vi "Hold to Floor_Save Sweep Data to csv.vi"(0 "Test Information":T2={"Exp Name"="Cold Switching", "Lot"="0233A", "Wafer"="15", "Die Type"="L22", "Die X "="6", "Die Y"="8", "Exp"="1", "Die X_Y"="8"}, 1 "Filepath":path, 5 "Date Cluster":T3, 7 "Selected Exp Settings":T5={"Floor_Sweep_Stop_V"=36.0, "Resistance Threshold"=1.0, "Floor_Sweep_Start_V"=36.0, "Floor_Sweep_Step_V"=1.0, "Roof_Sweep_Stop_V"=36.0, "Roof_Sweep_Start_V"=36.0, "Roof_Sweep_Step_V"=1.0, "Experiment Name"="", "Meas_Type"=[0, 2, 4]}, 9 "ks5080A_Meaurements":T4, 11 "Cal Measurements":T7 {"Port 3 Capacitance" format="%#_6p"; "Port 2 Capacitance" format="%#_6p"; "Port 1 Capacitance" format="%#_6p"}, 12 "Additional Data":T8, 13 "Time":dbl[](array[numeric]), 14 "Meas Type":string="QuickView_") -> ()   [LabVIEW 2013]
uses:
  Controls/Date Control.ctl
  Controls/Test Information.ctl
  Controls/Additional Data.ctl
  Controls/ks5080A_Measurements.ctl
  Controls/Individual User Inputs_MultiTest.ctl
  Controls/Test Selection.ctl
  Controls/ENA_Marker Measurements.ctl
  <vilib>/Utility/file.llb/Write To Spreadsheet File (string).vi
panel:
  in  "Tab Control":T1(tab)
  # "Calculation Settings"
  # "Test Settings"
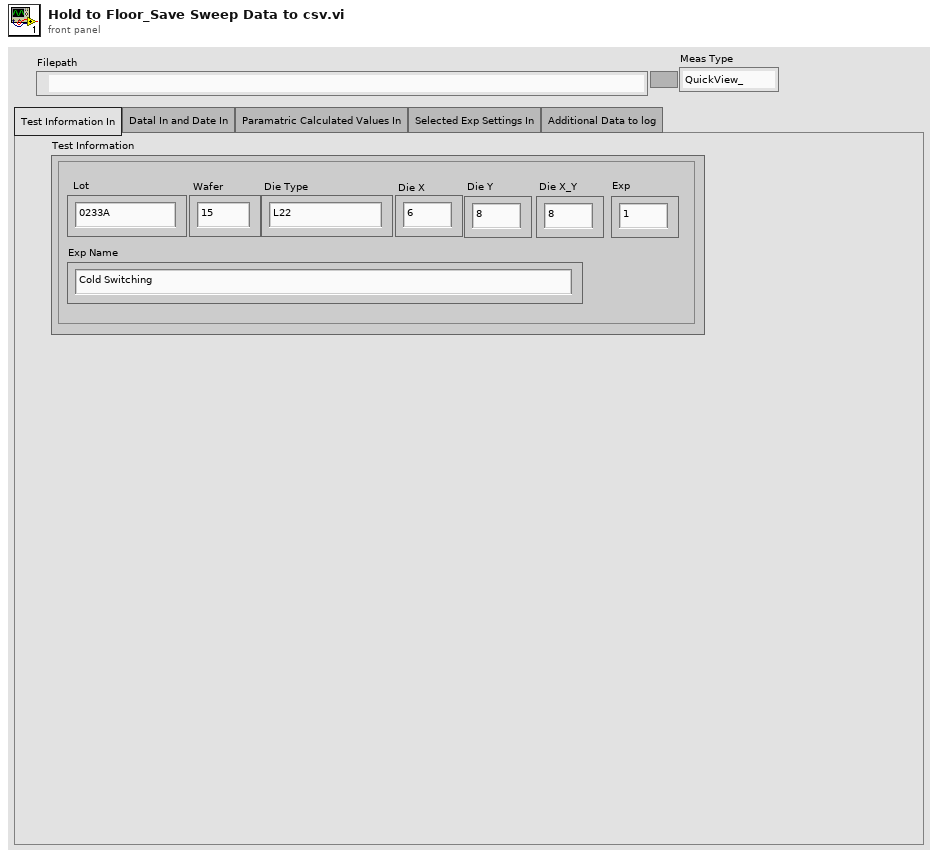
[diagram p1: front panel]
types:
  T1 = enum32{"Test Information In", "Datal In and Date In", "Paramatric Calculated Values In", "Selected Exp Settings In", "Additional Data to log"}
  T2 = typedef "Test Information.ctl" = cluster{"Exp Name":string, "Lot":string, "Wafer":string, "Die Type":string, "Die X ":string, "Die Y":string, "Exp":string, "Die X_Y":string}
  T3 = typedef "Date Control.ctl" = cluster{"Date":string, "Start Time":string, "Stop Time":string}
  T4 = typedef "ks5080A_Measurements.ctl" = cluster{"Bias_Sweep_Setting":dbl[], "Bias_voltage measurements":dbl[], "Bias_current measurements":dbl[], "P1_Capacitance":dbl[], "P2_Capacitance":dbl[], "DMM_Measurement_V":dbl[], "Contact_Source Current measurements":dbl[], "Contact_Sink Current measurements":dbl[], "Calculated_Resistance":dbl[], "P3_Capacitance":dbl[], "Port 1_S_parm":string[], "Port 2_S_parm":string[], "Port 3_S_parm":string[]}
  T5 = typedef "Individual User Inputs_MultiTest.ctl" = cluster{"Floor_Sweep_Stop_V":dbl, "Resistance Threshold":dbl, "Floor_Sweep_Start_V":dbl, "Floor_Sweep_Step_V":dbl, "Roof_Sweep_Stop_V":dbl, "Roof_Sweep_Start_V":dbl, "Roof_Sweep_Step_V":dbl, "Experiment Name":string, "Meas_Type":T6}
  T6 = typedef "Test Selection.ctl" = i32[]
  T7 = typedef "ENA_Marker Measurements.ctl" = cluster{"Port 1 Capacitance":dbl[], "Port 2 Capacitance":dbl[], "Port 3 Capacitance":dbl[], "Port 1_S_parm":string[], "Port 2_S_parm":string[], "Port 3_S_parm":string[]}
  T8 = typedef "Additional Data.ctl" = cluster{"P2_Capacitance_PostTest":dbl[], "P1_Capacitance _PostTest":dbl[], "P1_Capacitance_PreTest":dbl[], "P2_Capacitance_PreTest":dbl[]}
  T9 = enum16{"open", "replace", "create", "open or create", "replace or create", "replace or create with confirmation"}
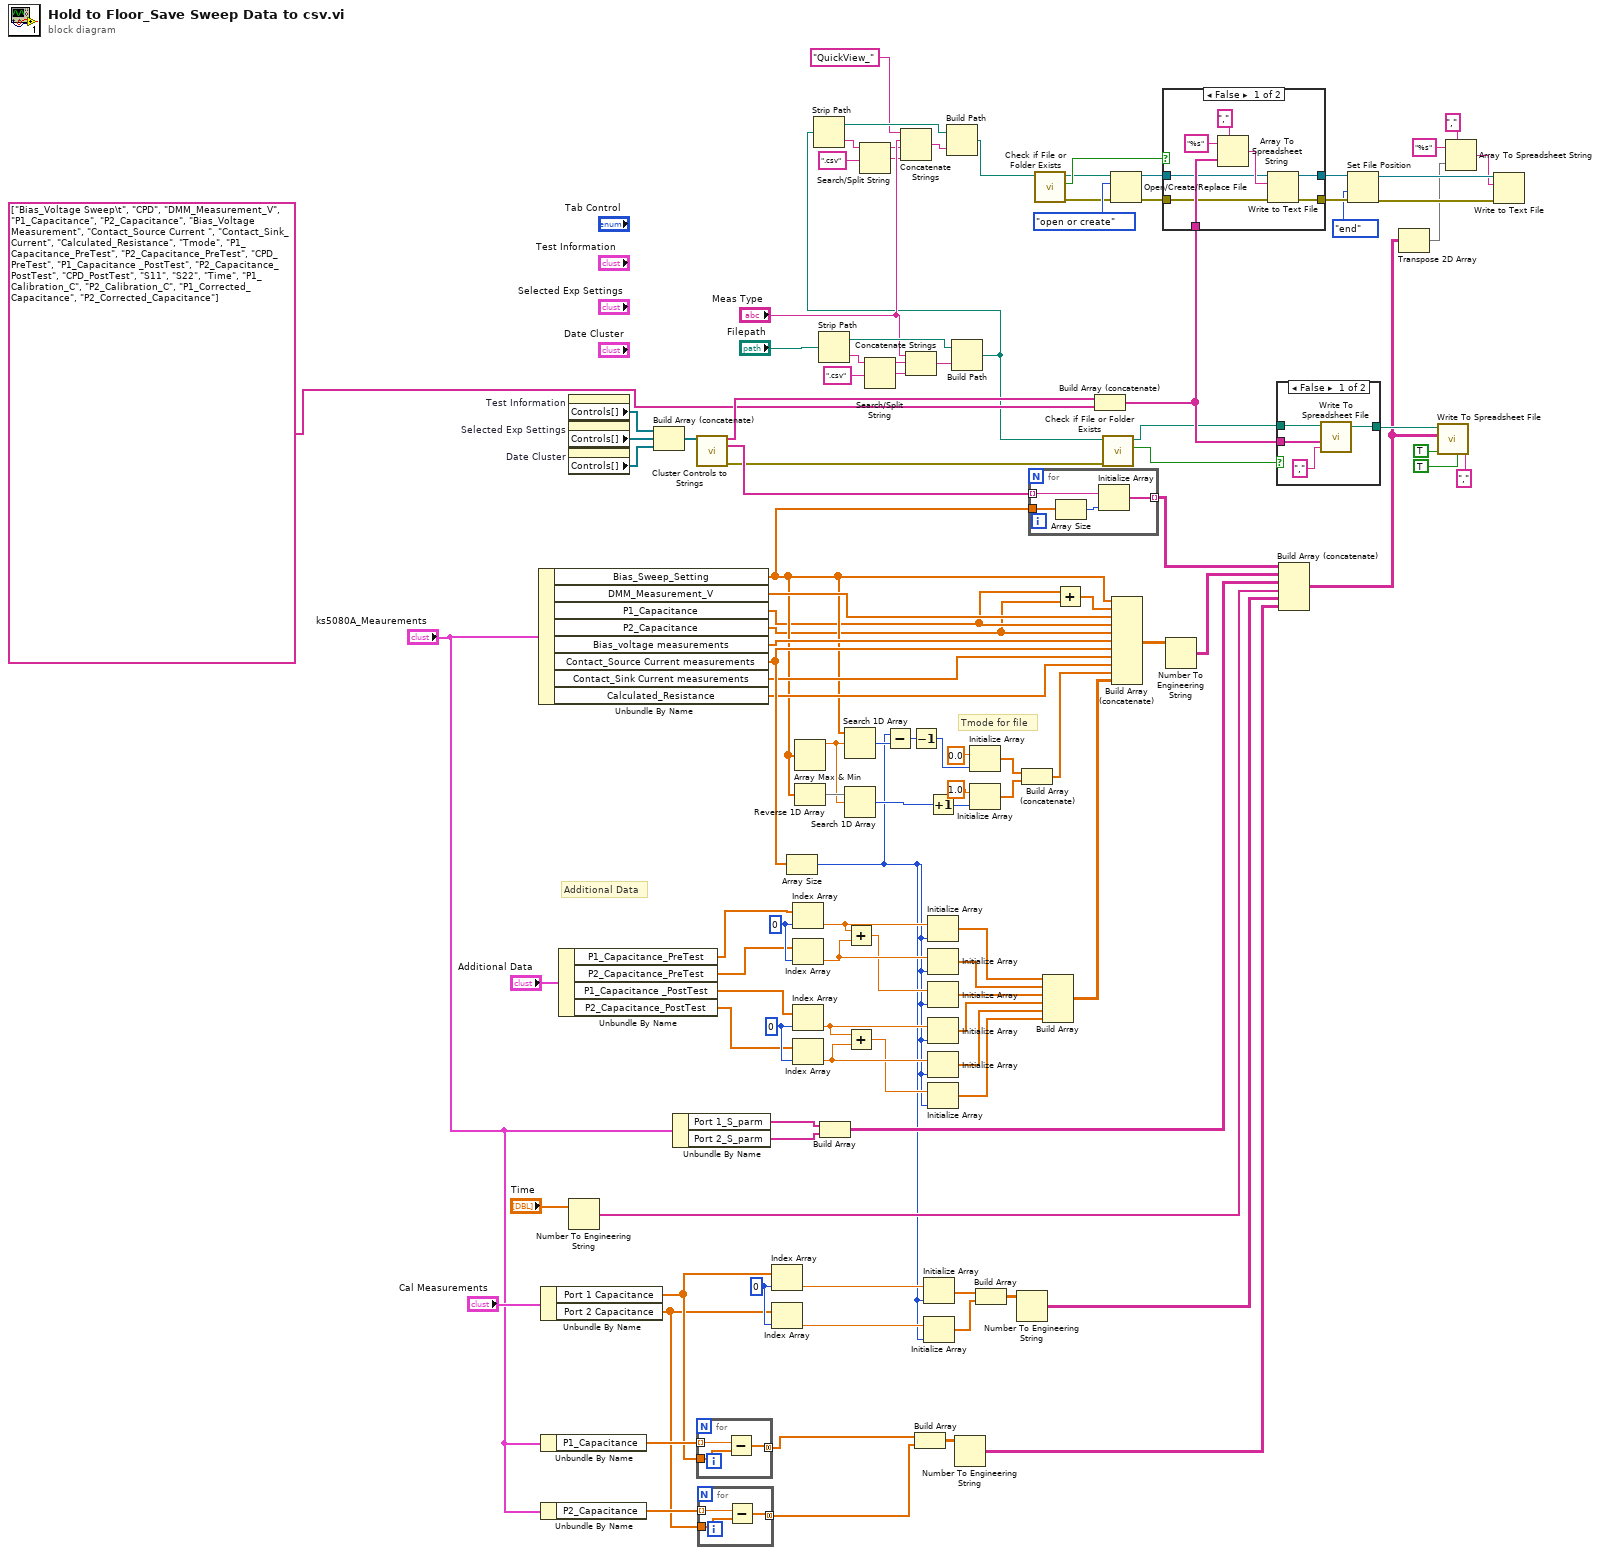
[diagram p0: block diagram]
diagram:
  w17 = 0 ("index")
  w98 = 0 ("index")
  w99 = 0 ("index")
  # "Tmode for file"
  # "Additional Data"
  n1 = Unbundle By Name("ks5080A_Meaurements") -> ("Bias_Sweep_Setting"=w23:dbl[], "DMM_Measurement_V"=w73:dbl[], "P1_Capacitance"=w21:dbl[], "P2_Capacitance"=w20:dbl[], "Bias_voltage measurements"=w72:dbl[], "Contact_Source Current measurements"=w71:dbl[], "Contact_Sink Current measurements"=w70:dbl[], "Calculated_Resistance"=w69:dbl[])
  n2 = Unbundle By Name("Cal Measurements") -> ("Port 1 Capacitance"=w5:dbl[], "Port 2 Capacitance"=w4:dbl[])
  n3 = Unbundle By Name("ks5080A_Meaurements") -> ("P1_Capacitance"=w11:dbl[])
  n4 = Unbundle By Name("ks5080A_Meaurements") -> ("P2_Capacitance"=w9:dbl[])
  n5 = Unbundle By Name("Additional Data") -> ("P1_Capacitance_PreTest"=w83:dbl[], "P2_Capacitance_PreTest"=w82:dbl[], "P1_Capacitance _PostTest"=w81:dbl[], "P2_Capacitance_PostTest"=w80:dbl[])
  n6 = property on="Test Information" class="Clust (strict)"() -> ("Controls[]"=w115:refnum<vi>[])  [unwired: 2 in, 2 out]
  n7 = property on="Selected Exp Settings" class="Clust (strict)"() -> ("Controls[]"=w38:refnum<vi>[])  [unwired: 2 in, 2 out]
  n8 = property on="Date Cluster" class="Clust (strict)"() -> ("Controls[]"=w113:refnum<vi>[])  [unwired: 2 in, 2 out]
  n9 = Number To Engineering String(4:"Time") -> (0:w36:string[])  [unwired: 3 in]
  n10 = Build Array (concatenate)(w115, w38, w113) -> (w114:refnum<vi>[])
  n11 = Unbundle By Name("ks5080A_Meaurements") -> ("Port 1_S_parm"=w68:string[], "Port 2_S_parm"=w67:string[])
  n12 = call "Cluster Controls to Strings.vi"("Controls[]"=w114) -> ("Control Labels"=w104:string[], "Control Values"=w112:string[], "Error Out"=w103:errorcluster)  [unwired: 12 in]
  n13 = for {
    tunnel: w11 -> [w118] mode=indexing
    tunnel: w5 -> [w117]
    tunnel: [w116] -> w10 mode=concatenating
    n14 = Subtract(x=w118, y=w117) -> (x-y=w116:dbl[])
  }
  n15 = for {
    tunnel: w9 -> [w121] mode=indexing
    tunnel: w4 -> [w120]
    tunnel: [w119] -> w8 mode=concatenating
    n16 = Subtract(x=w121, y=w120) -> (x-y=w119:dbl[])
  }
  n17 = Index Array(array=w5, index=w17) -> (element=w18:dbl)
  n18 = Index Array(array=w4, index=w17) -> (element=w16:dbl)
  n19 = Array Size(array=w71) -> (size(s)=w1:i32)
  n20 = Index Array(array=w83, index=w99) -> (element=w97:dbl)
  n21 = Index Array(array=w82, index=w99) -> (element=w96:dbl)
  n22 = Index Array(array=w81, index=w98) -> (element=w94:dbl)
  n23 = Index Array(array=w80, index=w98) -> (element=w93:dbl)
  n24 = Array Max & Min(array=w23) -> (max value=w30:dbl)  [unwired: 3 out]
  n25 = Reverse 1D Array(array=w23) -> (reversed array=w31:dbl[])
  n26 = Strip Path(path="Filepath") -> (stripped path=w76:path, name=w79:string)
  n27 = Build Array(w68, w67) -> (w66:string[][])
  n28 = Search 1D Array(1D array=w23, element=w30) -> (index of element=w29:i32)  [unwired: 1 in]
  n29 = Search 1D Array(1D array=w31, element=w30) -> (index of element=w26:i32)  [unwired: 1 in]
  n30 = Add(x=w97, y=w96) -> (x+y=w95:dbl)
  n31 = Add(x=w94, y=w93) -> (x+y=w92:dbl)
  n32 = Search/Split String(string=w79, search string/char (-)=".csv" ("search string")) -> (substring before match=w74:string, match + rest of string=w77:string)  [unwired: 1 in, 1 out]
  n33 = Subtract(x=w1, y=w29) -> (x-y=w28:i32)
  n34 = Concatenate Strings("Meas Type", w74, w77) -> (w75:string)
  n35 = Decrement(x=w28) -> (x-1=w27:i32)
  n36 = Build Array(w10, w8) -> (w7:dbl[][])
  n37 = Initialize Array(w18, w1) -> (w14:dbl[])
  n38 = Initialize Array(w16, w1) -> (w15:dbl[])
  n39 = Increment(x=w26) -> (x+1=w25:i32)
  n40 = Initialize Array(w97, w1) -> (w91:dbl[])
  n41 = Initialize Array(w96, w1) -> (w90:dbl[])
  n42 = Initialize Array(w95, w1) -> (w89:dbl[])
  n43 = Initialize Array(w94, w1) -> (w88:dbl[])
  n44 = Initialize Array(w93, w1) -> (w87:dbl[])
  n45 = Initialize Array(w92, w1) -> (w86:dbl[])
  n46 = Build Path(base path=w76, name or relative path=w75) -> (appended path=w19:path)
  n47 = Strip Path(path=w19) -> (stripped path=w57:path, name=w60:string)
  n48 = Search/Split String(string=w60, search string/char (-)=".csv" ("search string")) -> (substring before match=w55:string, match + rest of string=w58:string)  [unwired: 1 in, 1 out]
  n49 = Concatenate Strings("QuickView_" ("search string"), "Meas Type", w55, w58) -> (w56:string)
  n50 = Build Path(base path=w57, name or relative path=w56) -> (appended path=w42:path)
  n51 = Number To Engineering String(4:w7) -> (0:w2:string[][])  [unwired: 3 in]
  n52 = Initialize Array(0.0, w27) -> (w35:dbl[])
  n53 = Initialize Array(1.0, w25) -> (w32:dbl[])
  n54 = Build Array(w14, w15) -> (w13:dbl[][])
  n55 = Number To Engineering String(4:w13) -> (0:w3:string[][])  [unwired: 3 in]
  n56 = Build Array (concatenate)(w35, w32) -> (w24:dbl[])
  n57 = for {
    tunnel: w23 -> [w125]
    tunnel: w112 -> [w124] mode=indexing
    tunnel: [w122] -> w107 mode=indexing
    n58 = Array Size(array=w125) -> (size(s)=w123:i32)
    n59 = Initialize Array(w124, w123) -> (w122:string[])
  }
  n60 = call <vilib>:"Check if File or Folder Exists.vi"("path"=w42) -> ("error out"=w41:errorcluster, "file or folder exists?"=w40:bool, "dup path"=w39:path)  [unwired: 8 in]
  n61 = Build Array(w91, w90, w89, w88, w87, w86) -> (w85:dbl[][])
  n62 = Add(x=w21, y=w20) -> (x+y=w22:dbl[])
  n63 = Build Array (concatenate)(w104, string[] ["Bias_Voltage Sweep\t", "CPD", "DMM_Measurement_V", "P1_Capacitance", "P2_Capacitance", "Bias_Voltage Measurement", "Contact_Source Current ", "Contact_Sink_Current", "Calculated_Resistance", "Tmode", "P1_Capacitance_PreTest", "P2_Capacitance_PreTest", "CPD_PreTest", "P1_Capacitance _PostTest", "P2_Capacitance_PostTest", "CPD_PostTest", "S11", "S22", "Time", "P1_Calibration_C", "P2_Calibration_C", "P1_Corrected_Capacitance", "P2_Corrected_Capacitance"]) -> (w101:string[])
  n64 = call <vilib>:"Check if File or Folder Exists.vi"("error in (no error)"=w103, "path"=w19) -> ("file or folder exists?"=w102:bool, "dup path"=w62:path)  [unwired: 7 in, 1 out]
  n65 = Open/Create/Replace File(file path (use dialog)=w39, error in=w41, operation (0:open)=T9."open or create") -> (refnum out=w54:refnum<file>, error out=w53:errorcluster)  [unwired: 3 in, 1 out]
  n66 = Build Array (concatenate)(w23, w22, w73, w21, w20, w72, w71, w70, w69, w24, w85) -> (w105:dbl[][])
  n67 = case shown="False" w40 {
    tunnel: w101 -> [w131 _]
    tunnel: w54 -> [w129 w135]
    tunnel: w53 -> [w128 w134]
    tunnel: [w127 w134] -> w51
    tunnel: [w126 w135] -> w52
    frame False {
      n68 = Array To Spreadsheet String(delimiter (Tab)="," ("delimiter (\\t)"), array=w131, 3:"%s" ("format string")) -> (spreadsheet string=w130:string)
      n69 = Write to Text File(file (use dialog)=w129, text=w130, error in=w128) -> (refnum out=w126:refnum<file>, error out=w127:errorcluster)  [unwired: 1 in, 1 out]
    }
    frame True {
    }
  }
  n70 = Number To Engineering String(4:w105) -> (0:w106:string[][])  [unwired: 3 in]
  n71 = case shown="False" w102 {
    tunnel: w62 -> [w139 w140]
    tunnel: w101 -> [w138 _]
    tunnel: [w136 w140] -> w111
    frame False {
      n72 = call-poly <vilib>:"Write To Spreadsheet File.vi"("delimiter (\\t)"="," ("delimiter (\\t)"), "1D data"=w138, "file path (dialog if empty)"=w139) -> ("new file path (Not A Path if cancelled)"=w136:path)  [unwired: 5 in]
    }
    frame True {
    }
  }
  n73 = Build Array (concatenate)(w107, w106, w66, w36, w3, w2) -> (w100:string[][])
  n74 = Set File Position(refnum=w52, from (0:start)=enum16{"start", "end", "current"}."end", error in=w51) -> (refnum out=w46:refnum<file>, error out=w47:errorcluster)  [unwired: 1 in]
  n75 = Transpose 2D Array(2D array=w100) -> (transposed array=w44:string[][])
  n76 = call-poly <vilib>:"Write To Spreadsheet File.vi"("delimiter (\\t)"="," ("delimiter (\\t)"), "transpose? (no:F)"=TRUE, "append to file? (new file:F)"=TRUE, "2D data"=w100, "file path (dialog if empty)"=w111) -> ()  [unwired: 3 in, 1 out]
  n77 = Array To Spreadsheet String(delimiter (Tab)="," ("delimiter (\\t)"), array=w44, 3:"%s" ("format string")) -> (spreadsheet string=w45:string)
  n78 = Write to Text File(file (use dialog)=w46, text=w45, error in=w47) -> ()  [unwired: 1 in, 3 out]
